vi "sc5511a_open_device.vi"(0 "Device SN String":string="10000AAA", 5 "error in (no error)":errorcluster) -> (14 "deviceHandle":u32 format="%.0x", 19 "error out":errorcluster)   [LabVIEW 2010]
uses:
  sc5511a.dll
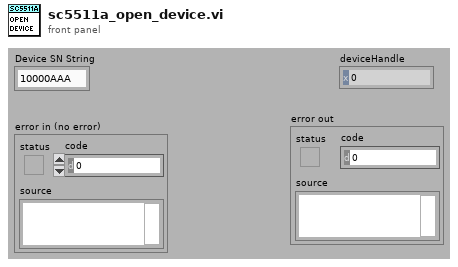
[diagram p1: front panel]
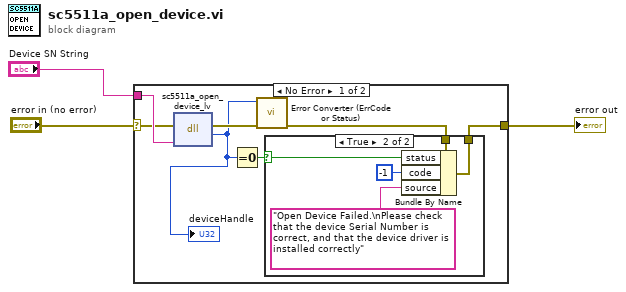
[diagram p0: block diagram]
diagram:
  n1 = case shown="No Error" "error in (no error)" {
    selector: "error in (no error)" -> [w4 w17]
    tunnel: [w7 w17] -> w2
    tunnel: "Device SN String" -> [w9 _]
    frame No Error {
      n2 = dll-call lib="sc5511a.dll" fn="sc5511a_open_device_lv"(error in=w4, "SerialNumber"=w9) -> (error out=w10:errorcluster, "devHandle"=w5:u32)  [unwired: 3 in, 1 out]
      "deviceHandle" <- w5
      n3 = Equal To 0?(x=w5) -> (x = 0?=w6:bool)
      n4 = call "Error Converter (ErrCode or Status).vi"("error in (no error)"=w10, "error code"=w5) -> ("error out"=w8:errorcluster)  [unwired: 9 in]
      n5 = case shown="True" w6 {
        selector: w6 -> [_ w13]
        tunnel: w8 -> [w11 w16]
        tunnel: [w11 w15] -> w7
        frame False {
        }
        frame True {
          n6 = Bundle By Name(cluster=w16, "status"=w13, "code"=-1, "source"="Open Device Failed.\nPlease check that the device Serial Number is correct, and that the device driver is installed correctly") -> (w15:errorcluster)
        }
      }
    }
    frame Error {
    }
  }
  "error out" <- w2
